vi "ziExample-Module-PIDAdvisor.vi"() -> ()   [LabVIEW 2009]
doc: "Control a Zurich instrument device via the LabOne Labview API. \nRequirements: Zurich Instruments HF2 +MF or UHFLI +MF \nPlease connect Signal input 1 and Signall Output 1.\nThis example shows how to configure a PID to regulate the output amplitude in order to achieve a constant input amplitude.\nThis example suggests a PID configuration via the PID advisor.\n\n© Zurich Instruments AG, www.zhinst.com"
uses:
  <instrlib>/Zurich Instruments LabOne/Public/ziTypeHandle.ctl
  <instrlib>/Zurich Instruments LabOne/Public/Modules/ziTypeModEnum.ctl
  <instrlib>/Zurich Instruments LabOne/Public/Modules/ziModSetValueBinary.vi
  <instrlib>/Zurich Instruments LabOne/Public/Configure/ziSetValueDouble.vi
  <instrlib>/Zurich Instruments LabOne/Public/Configure/ziSetValueDoubleArray.vi
  <instrlib>/Zurich Instruments LabOne/Public/Configure/ziGetValueString.vi
  <instrlib>/Zurich Instruments LabOne/Public/Modules/ziModSetValueDouble.vi
  <instrlib>/Zurich Instruments LabOne/Public/Modules/ziModSetValueDoubleArray.vi
  <instrlib>/Zurich Instruments LabOne/Public/Modules/ziModGetDoubleData.vi
  <instrlib>/Zurich Instruments LabOne/Public/Modules/ziModGetAdvisorData.vi
  <instrlib>/Zurich Instruments LabOne/Zurich Instruments LabOne.lvlib
panel:
  out "VALUE":dbl(graph)
  out "PID SHIFT":dbl(graph)
  out "demod/timeconstant":dbl
  out "Error Out":errorcluster
  out "Handle Out":T1 {"Handle" format="0x%08x"; "Conn" format="0x%08x"}
  in  "Calculate":bool
  in  "stop":bool
  out "PID ERROR":dbl(graph)
  in  "Address":string="DEV"
  in  "bw":dbl=100.0 caption="target BW (Hz)"
  in  "Mode":dbl(ring)=3.0 items=["P"=1.0, "I"=2.0, "PI"=3.0, "PID"=7.0, "PIDF"=15.0]
  out "i":dbl caption="I"
  out "p":dbl caption="P"
  out "dlimittimeconstant":dbl
  out "rate":dbl caption="Rate (Hz)"
  out "d":dbl caption="D"
  out "Step Response":cluster{"grid":dbl[], "r_avg":dbl[]}(graph)
  out "Bode Gain":cluster{"grid":dbl[], "r_avg":dbl[]}(graph)
  out "Bode Phase":cluster{"grid":dbl[], "r_avg":dbl[]}(graph)
  out "Selected Device":string
  # "ziExample-Module-PIDAdvisor.vi\nRequirements: UHFLI, HF2, MFLI +PID\nsee block diagram for VI description"
  # "Tested Devices:\n- UHFLI+PID \n- HF2+PID\n- MFLI+PID"
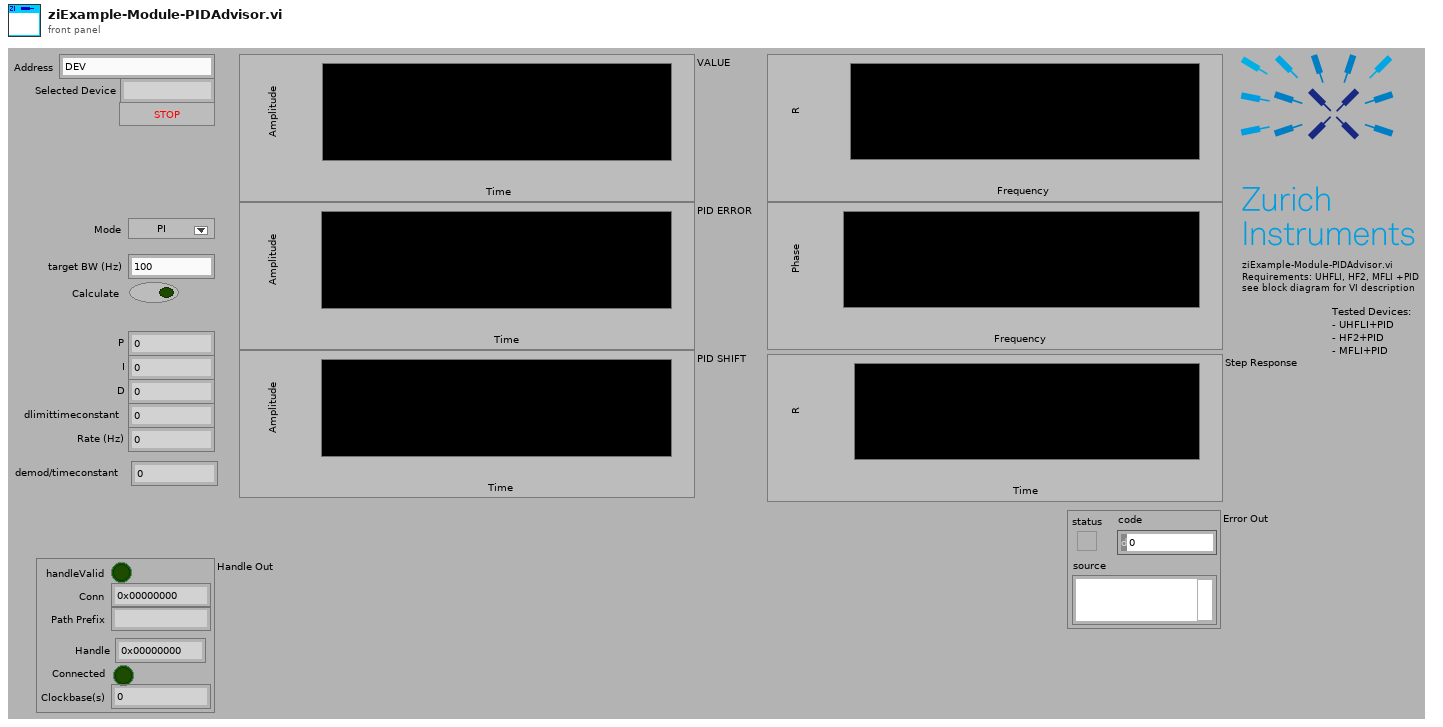
[diagram p1: front panel]
types:
  T1 = typedef "Zurich Instruments LabOne.lvlib/ziTypeHandle.ctl" = cluster{"handleValid":bool, "Conn":u64, "Path Prefix":string, "Handle":u64, "Connected":bool, "Clockbase(s)":dbl}
  T2 = typedef "Zurich Instruments LabOne.lvlib/ziTypeModEnum.ctl" = u16
  T3 = typedef "Zurich Instruments LabOne.lvlib/ziTypeModHandle.ctl" = cluster{"handleValid":bool, "Conn":u64, "ModHandle":u64, "moduleID":string, "Path Prefix":string}
  T4 = typedef "Zurich Instruments LabOne.lvlib/ziTypeModResults.ctl" = cluster{"PathArray":string[], "ValueType":T5, "NoOfResults":u64, "ziGenericHeader":T6[]}
  T5 = typedef "Zurich Instruments LabOne.lvlib/ziTypePollType.ctl" = enum16{"NONE", "DOUBLE_DATA", "INTEGER_DATA", "DEMOD_SAMPLE", "SCOPE_WAVE_HF2", "AUXIN_SAMPLE", "DIO_SAMPLE", "BYTE_ARRAY", "PWA_WAVE", "9", "10", "11", "12", "13", "14", "15", "TREE_CHANGE_DEPRI", "17", "ERROR", "19", "20", "21", "22", "23", "24", "25", "26", "27", "28", "29", "30", "31", "DOUBLE_DATA_TS", "INTEGER_DATA_TS", "34", "SCOPE_WAVE", "SCOPE_WAVE_EX", "37", "BYTE_ARRAY_TS", "39", "40", "41", "42", "43", "44", "45", "CNT_DATA", "47", "TREE_CHANGE", "49", "50", "51", "52", "53", "54", "55", "56", "57", "58", "59", "60", "61", "62", "63", "SWEEPER_DATA", "SPECTRUM_DATA", "ADVISOR_DATA", "VECTOR_DATA", "IMP_DATA"}
  T6 = typedef "Zurich Instruments LabOne.lvlib/ziTypeModGenericHeader.ctl" = cluster{"HeaderType":enum8{"HEADER_TYPE_NONE", "HEADER_TYPE_SWTRIGGER", "HEADER_TYPE_SWEEPER"}, "SampleFormat":u8, "SystemTime":timestamp, "CreatedTimeStamp":u64, "ChangedTimeStamp":u64, "Flags":u32, "ChunkSizeBytes":u64, "Name":string, "Status":u32, "GroupIndex":u32, "Color":u32, "ActiveRow":u32, "TriggerNumber":u64, "GridRows":u32, "GridCols":u32, "GridMode":u32, "GridOperation":u32, "GridDirection":u32, "GridRepetitions":u32, "GridColDelta":dbl, "GridColOffset":dbl, "GridRowDelta":dbl, "GridRowOffset":dbl, "Bandwidth":dbl, "Center":dbl, "Nenbw":dbl}
  T7 = typedef "Zurich Instruments LabOne.lvlib/ziTypeModAdvisorWave.ctl" = cluster{"timestamp":u64, "sampleCount":u64, "flags":u8, "sampleFormat":u8, "grid":dbl[], "x":dbl[], "y":dbl[]}
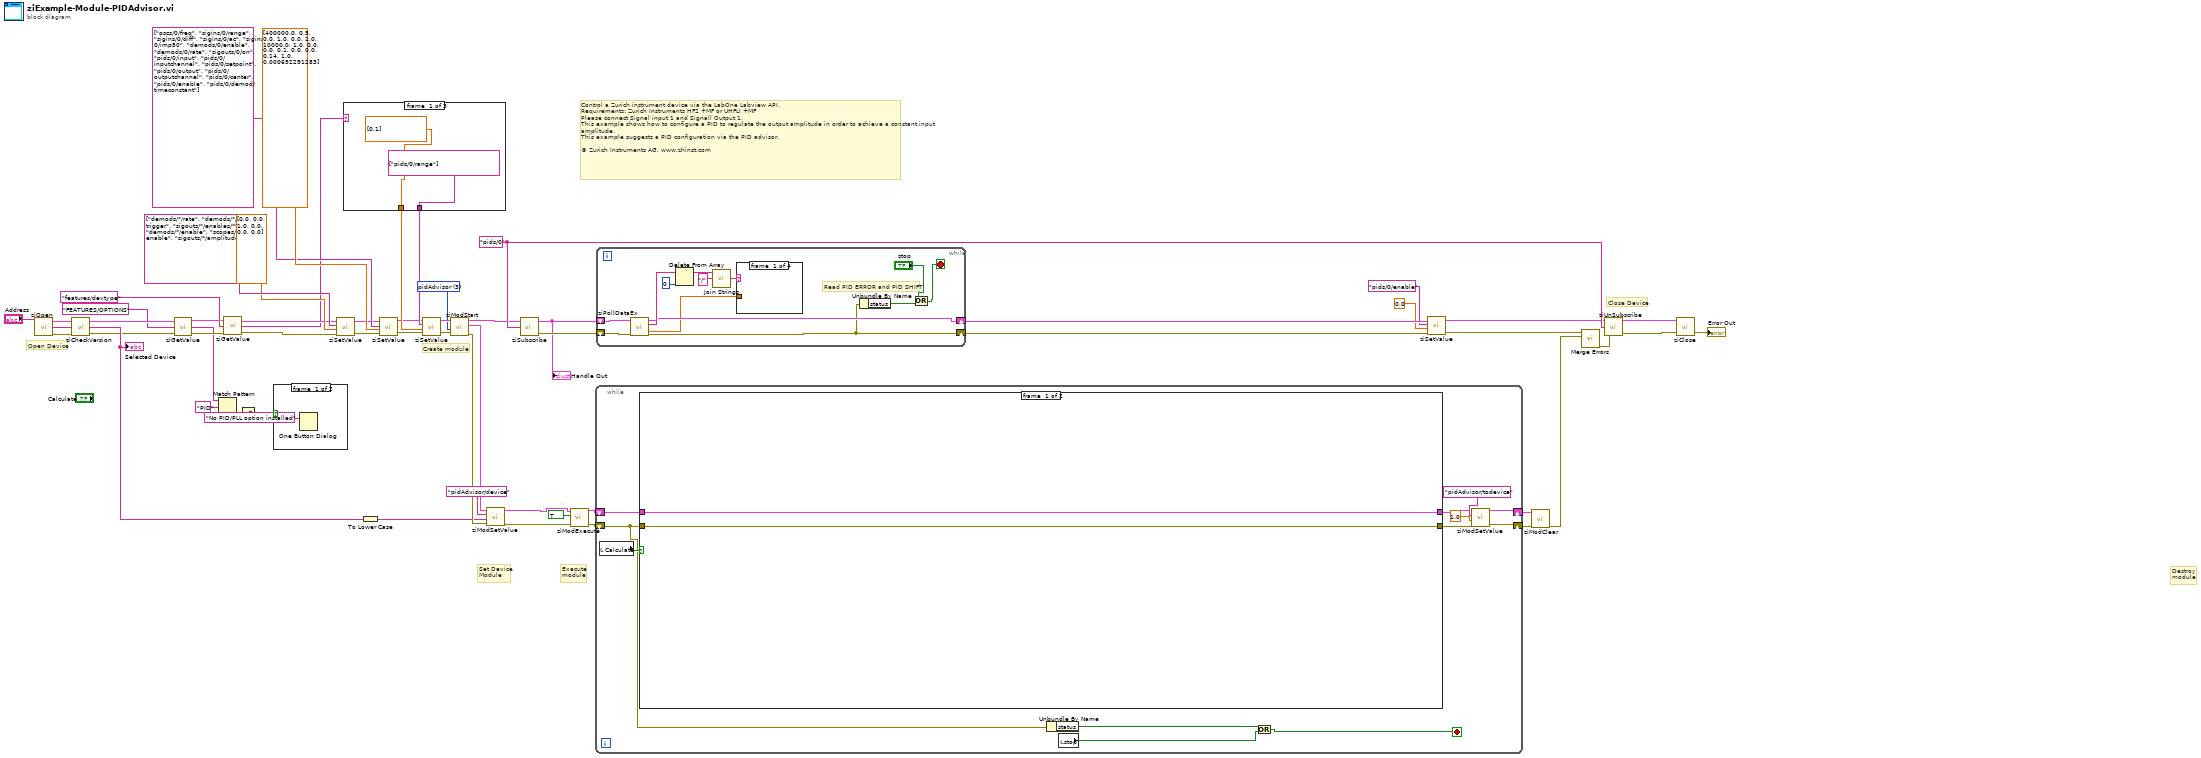
[diagram p0: block diagram]
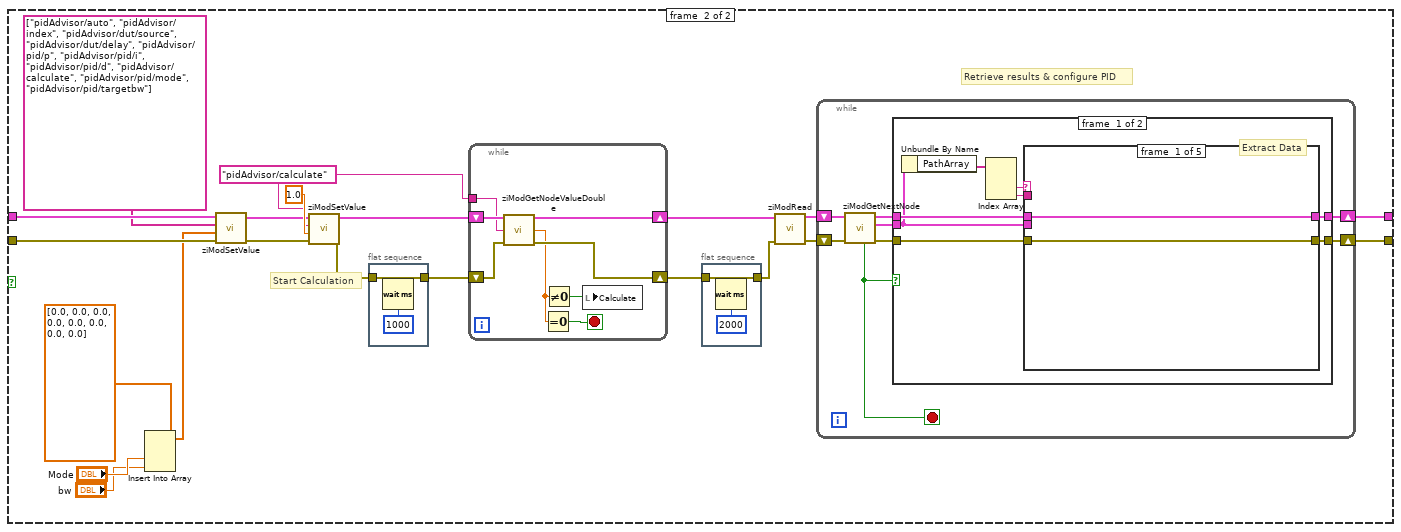
[diagram p3: hidden frame]
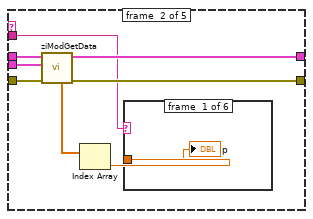
[diagram p4: hidden frame]
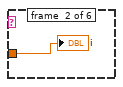
[diagram p5: hidden frame]
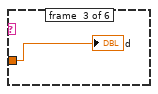
[diagram p6: hidden frame]
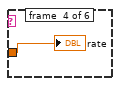
[diagram p7: hidden frame]
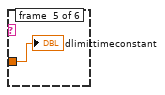
[diagram p8: hidden frame]
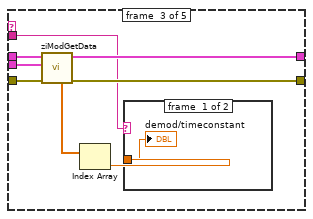
[diagram p10: hidden frame]
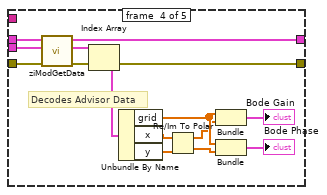
[diagram p12: hidden frame]
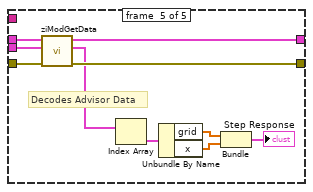
[diagram p13: hidden frame]
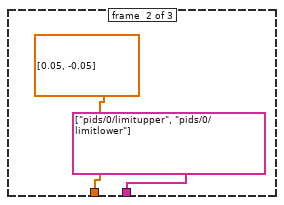
[diagram p15: hidden frame]
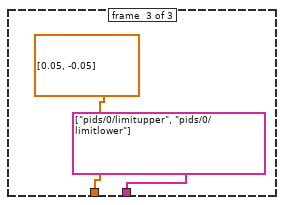
[diagram p16: hidden frame]
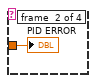
[diagram p17: hidden frame]
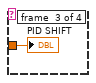
[diagram p18: hidden frame]
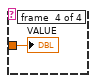
[diagram p19: hidden frame]
diagram:
  w15 = T2 3 items=["sweep", "scopeModule", "dataAcquisitionModule", "pidAdvisor", "awgModule", "impedanceModule", "multiDeviceSyncModule", "zoomFFT", "trigger", "deviceSettings", "record"] ("module Id")
  w38 = "pids/0" ("Path ()")
  # "Control a Zurich instrument device via the LabOne Labview API. \nRequirements: Zurich Instruments HF2 +MF or UHFLI +MF \nPlease connect Signal input 1 and Signall Output 1.\nThis example shows how to configure a PID to regulate the output amplitude in order to achieve a constant input amplitude.\nThis example suggests a PID configuration via the PID advisor.\n\n© Zurich Instruments AG, www.zhinst.com"
  # "Execute\nmodule"
  # "Set Device\nModule"
  # "Destroy\nmodule"
  # "Create module"
  # "Close Device"
  # "Open Device"
  n1 = call <instrlib>:"ziOpen.vi"("Address"="Address") -> ("Error Out"=w16:errorcluster, "Selected Device"=w36:string, "HandleOut"=w17:T1)  [unwired: 1 in, 2 out]
  "Selected Device" <- w36
  n2 = call <instrlib>:"ziCheckVersion.vi"("Handle In"=w17, "Error In"=w16) -> ("Handle Out"=w10:T1, "Error Out"=w9:errorcluster)  [unwired: 11 in, 1 out]
  n3 = call-poly <instrlib>:"ziGetValue.vi"("error in"=w9, "Path"="FEATURES/OPTIONS", "Handle In"=w10) -> ("error out"=w12:errorcluster, "Value"=w7:string, "Handle Out"=w11:T1)
  n4 = Match Pattern(string=w7, regular expression="PID") -> (offset past match=w13:i32)  [unwired: 1 in, 3 out]
  n5 = call-poly <instrlib>:"ziGetValue.vi"("error in"=w12, "Path"="features/devtype", "Handle In"=w11) -> ("error out"=w20:errorcluster, "Value"=w18:string, "Handle Out"=w21:T1)
  n6 = Greater Or Equal To 0?(x=w13) -> (x >= 0?=w1:bool)
  n7 = case shown="True" w1 {
    frame #0 {
      n8 = One Button Dialog(message="No PID/PLL option installed") -> ()  [unwired: 1 in, 1 out]
    }
    frame #1 {
    }
  }
  n9 = call-poly <instrlib>:"ziSetValue.vi"("Error In"=w20, "Values"=dbl[] [0.0, 0.0, 1.0, 0.0, 0.0, 0.0], "Paths"=string[] ["demods/*/rate", "demods/*/trigger", "sigouts/*/enables/*", "demods/*/enable", "scopes/*/enable", "sigouts/*/amplitudes/*"], "Handle In"=w21) -> ("Error Out"=w22:errorcluster, "Handle Out"=w23:T1)  [unwired: 1 in]
  n10 = case shown="\"MFIA\", \"MFLI\"" w18 {
    tunnel: [dbl[] [0.1] dbl[] [0.05, -0.05] dbl[] [0.05, -0.05]] -> w43
    tunnel: [string[] ["pids/0/range"] string[] ["pids/0/limitupper", "pids/0/limitlower"] string[] ["pids/0/limitupper", "pids/0/limitlower"]] -> w42
    frame #0 {
    }
    frame #1 {
    }
    frame #2 {
    }
  }
  n11 = To Lower Case(string=w36) -> (all lower case string=w35:string)
  n12 = call-poly <instrlib>:"ziSetValue.vi"("Error In"=w22, "Values"=dbl[] [400000.0, 0.5, 0.0, 1.0, 0.0, 1.0, 10000.0, 1.0, 0.0, 0.0, 0.1, 0.0, 0.0, 0.14, 1.0, 0.000692291283], "Paths"=string[] ["oscs/0/freq", "sigins/0/range", "sigins/0/diff", "sigins/0/ac", "sigins/0/imp50", "demods/0/enable", "demods/0/rate", "sigouts/0/on", "pids/0/input", "pids/0/inputchannel", "pids/0/setpoint", "pids/0/output", "pids/0/outputchannel", "pids/0/center", "pids/0/enable", "pids/0/demod/timeconstant"], "Handle In"=w23) -> ("Error Out"=w27:errorcluster, "Handle Out"=w28:T1)  [unwired: 1 in]
  n13 = call-poly <instrlib>:"ziSetValue.vi"("Error In"=w27, "Values"=w43, "Paths"=w42, "Handle In"=w28) -> ("Error Out"=w55:errorcluster, "Handle Out"=w56:T1)  [unwired: 1 in]
  n14 = call <instrlib>:"ziModStart.vi"("Error In"=w55, "module Id"=w15, "Handle In"=w56) -> ("Error Out"=w46:errorcluster, "ModHandle Out"=w52:T3, "Handle Out"=w19:T1)  [unwired: 6 in]
  n15 = call-poly <instrlib>:"ziModSetValue.vi"("Error In"=w46, "Data"=w35, "Path"="pidAdvisor/device", "ModHandle In"=w52) -> ("Error Out"=w5:errorcluster, "ModHandle Out"=w6:T3)  [unwired: 6 in]
  n16 = call <instrlib>:"ziSubscribe.vi"("Path ()"=w38, "Handle In"=w19) -> ("error out"=w53:errorcluster, "Handle Out"=w47:T1)  [unwired: 2 in]
  "Handle Out" <- w47
  n17 = call <instrlib>:"ziModExecute.vi"("Error In"=w5, "Modal (F)"=TRUE ("Modal"), "ziModHandle In"=w6) -> ("Error Out"=w51:errorcluster, "ziModHandle Out"=w48:T3)  [unwired: 5 in, 1 out]
  n18 = while {
    shift-right: [w70] -> w3
    shift-left: w48 -> [w75]
    shift-right: [w69] -> w4
    shift-left: w51 -> [w67]
    stop <- w64 stop-if-true
    n19 = local read "Calculate"() -> (w74:bool)
    n20 = case shown="True" w74 {
      tunnel: w75 -> [w76 w92]
      tunnel: w67 -> [w77 w93]
      tunnel: [w77 w85] -> w68
      tunnel: [w76 w86] -> w71
      frame #0 {
      }
      frame #1 {
        w79 = "pidAdvisor/calculate" ("Path")
        # "Extract Data"
        # "Retrieve results & configure PID"
        # "Start Calculation"
        n21 = Insert Into Array(array=dbl[] [0.0, 0.0, 0.0, 0.0, 0.0, 0.0, 0.0, 0.0], new element #1="Mode", new element #2="bw") -> (w80:dbl[])  [unwired: 1 in]
        n22 = call-poly <instrlib>:"ziModSetValue.vi"("Error In"=w93, "Values"=w80, "Paths"=string[] ["pidAdvisor/auto", "pidAdvisor/index", "pidAdvisor/dut/source", "pidAdvisor/dut/delay", "pidAdvisor/pid/p", "pidAdvisor/pid/i", "pidAdvisor/pid/d", "pidAdvisor/calculate", "pidAdvisor/pid/mode", "pidAdvisor/pid/targetbw"], "ModHandle In"=w92) -> ("Error Out"=w78:errorcluster, "ModHandle Out"=w81:T3)  [unwired: 6 in]
        n23 = call-poly <instrlib>:"ziModSetValue.vi"("Error In"=w78, "Value"=1.0, "Path"=w79, "ModHandle In"=w81) -> ("Error Out"=w91:errorcluster, "ModHandle Out"=w96:T3)  [unwired: 6 in]
        n24 = flat-sequence {
          tunnel: [w102] -> w90
          tunnel: w91 -> [w102]
          frame #0 {
            n25 = Wait (ms)(milliseconds to wait=u32 1000) -> ()  [unwired: 1 out]
          }
        }
        n26 = while {
          shift-right: [w172] -> w97
          shift-left: w96 -> [w175]
          shift-right: [w173] -> w88
          shift-left: w90 -> [w176]
          tunnel: w79 -> [w174]
          stop <- w171 stop-if-true
          n27 = call <instrlib>:"ziModGetNodeValueDouble.vi"("ModHandle In"=w175, "Path"=w174, "error in"=w176) -> ("ModHandle Out"=w172:T3, "Value"=w169:dbl, "error out"=w173:errorcluster)  [unwired: 10 in]
          n28 = Equal To 0?(x=w169) -> (x = 0?=w171:bool)
          n29 = Not Equal To 0?(x=w169) -> (x != 0?=w170:bool)
          n30 = local write "Calculate"(w170) -> ()
        }
        n31 = flat-sequence {
          tunnel: w88 -> [w99]
          tunnel: [w99] -> w87
          frame #0 {
            n32 = Wait (ms)(milliseconds to wait=u32 2000) -> ()  [unwired: 1 out]
          }
        }
        n33 = call <instrlib>:"ziModRead.vi"("error in"=w87, "ziModHandle In"=w97) -> ("error out"=w94:errorcluster, "ziModHandle Out"=w95:T3)  [unwired: 8 in]
        n34 = while {
          shift-right: [w104] -> w86
          shift-left: w95 -> [w109]
          shift-right: [w103] -> w85
          shift-left: w94 -> [w110]
          stop <- w105 stop-if-true
          n35 = call <instrlib>:"ziModGetNextNode.vi"("Error In"=w110, "ModHandle In"=w109) -> ("Error Out"=w107:errorcluster, "ModResults"=w106:T4, "ModHandle Out"=w108:T3, "NoData"=w105:bool)  [unwired: 6 in]
          n36 = case shown="False" w105 {
            tunnel: w108 -> [w118 w168]
            tunnel: w107 -> [w117 w167]
            tunnel: w106 -> [w114 _]
            tunnel: [w116 w168] -> w104
            tunnel: [w115 w167] -> w103
            frame #0 {
              n37 = Unbundle By Name(w114) -> ("PathArray"=w113:string[])
              n38 = Index Array(array=w113) -> (element #2=w111:string, element #3=w112:string)  [unwired: 3 in, 1 out]
              n39 = case shown="Default" w111 {
                tunnel: w118 -> [w120 w128 w141 w155 w165]
                tunnel: w114 -> [_ w127 w140 w156 w166]
                tunnel: w117 -> [w119 w126 w139 w154 w164]
                tunnel: [w119 w123 w136 w153 w163] -> w115
                tunnel: [w120 w125 w138 w152 w162] -> w116
                tunnel: w112 -> [_ w122 w135 _ _]
                frame #0 {
                }
                frame #1 {
                  n40 = call-poly <instrlib>:"ziModGetData.vi"("Error In"=w126, "ModResults"=w127, "ModHandle In"=w128) -> ("Error Out"=w123:errorcluster, "ModHandle Out"=w125:T3, "Value"=w121:dbl[])  [unwired: 4 in, 2 out]
                  n41 = Index Array(array=w121) -> (element=w124:dbl)  [unwired: 1 in]
                  n42 = case shown="\"d\"" w122 {
                    tunnel: w124 -> [w129 w130 w131 w132 w133 _]
                    frame #0 {
                      "p" <- w129
                    }
                    frame #1 {
                      "i" <- w130
                    }
                    frame #2 {
                      "d" <- w131
                    }
                    frame #3 {
                      "rate" <- w132
                    }
                    frame #4 {
                      "dlimittimeconstant" <- w133
                    }
                    frame #5 {
                    }
                  }
                }
                frame #2 {
                  n43 = call-poly <instrlib>:"ziModGetData.vi"("Error In"=w139, "ModResults"=w140, "ModHandle In"=w141) -> ("Error Out"=w136:errorcluster, "ModHandle Out"=w138:T3, "Value"=w134:dbl[])  [unwired: 4 in, 2 out]
                  n44 = Index Array(array=w134) -> (element=w137:dbl)  [unwired: 1 in]
                  n45 = case shown="\"timeconstant\"" w135 {
                    tunnel: w137 -> [w142 _]
                    frame #0 {
                      "demod/timeconstant" <- w142
                    }
                    frame #1 {
                    }
                  }
                }
                frame #3 {
                  # "Decodes Advisor Data"
                  n46 = call-poly <instrlib>:"ziModGetData.vi"("Error In"=w154, "ModResults"=w156, "ModHandle In"=w155) -> ("Error Out"=w153:errorcluster, "AdvisorData Out"=w150:T7[], "ModHandle Out"=w152:T3)  [unwired: 6 in]
                  n47 = Index Array(array=w150) -> (element=w151:T7)  [unwired: 1 in]
                  n48 = Unbundle By Name(w151) -> ("grid"=w147:dbl[], "x"=w143:dbl[], "y"=w144:dbl[])
                  n49 = Re/Im To Polar(2:w144, 3:w143) -> (0:w145:dbl[], 1:w146:dbl[])
                  n50 = Bundle("grid"=w147, w146) -> (→"Bode Gain":cluster{"grid":dbl[], dbl[]})  [unwired: 1 in]
                  n51 = Bundle("grid"=w147, w145) -> (→"Bode Phase":cluster{"grid":dbl[], dbl[]})  [unwired: 1 in]
                }
                frame #4 {
                  # "Decodes Advisor Data"
                  n52 = call-poly <instrlib>:"ziModGetData.vi"("Error In"=w164, "ModResults"=w166, "ModHandle In"=w165) -> ("Error Out"=w163:errorcluster, "AdvisorData Out"=w160:T7[], "ModHandle Out"=w162:T3)  [unwired: 6 in]
                  n53 = Index Array(array=w160) -> (element=w161:T7)  [unwired: 1 in]
                  n54 = Unbundle By Name(w161) -> ("grid"=w159:dbl[], "x"=w158:dbl[])
                  n55 = Bundle("grid"=w159, "x"=w158) -> (→"Step Response":cluster{"grid":dbl[], "x":dbl[]})  [unwired: 1 in]
                }
              }
            }
            frame #1 {
              (unwired) FALSE
            }
          }
        }
      }
    }
    n56 = Unbundle By Name(w67) -> ("status"=w66:bool)
    n57 = local read "stop"() -> (w65:bool)
    n58 = Or(x=w66, y=w65) -> (x .or. y?=w64:bool)
    n59 = call-poly <instrlib>:"ziModSetValue.vi"("Error In"=w68, "Value"=1.0, "Path"="pidAdvisor/todevice", "ModHandle In"=w71) -> ("Error Out"=w69:errorcluster, "ModHandle Out"=w70:T3)  [unwired: 6 in]
  }
  n60 = while {
    shift-right: [w182] -> w33
    shift-left: w47 -> [w189]
    shift-right: [w180] -> w34
    shift-left: w53 -> [w188]
    stop <- w177 stop-if-true
    # "Read PID ERROR and PID SHIFT"
    n61 = call <instrlib>:"ziPollDataEx.vi"("error in"=w188, "Handle In"=w189) -> ("error out"=w180:errorcluster, "PathArray"=w186:string[], "Handle Out"=w182:T1, "Value Double"=w181:dbl)  [unwired: 2 in, 4 out]
    n62 = Delete From Array(array=w186, index=0) -> (array with subset deleted=w185:string[])  [unwired: 1 in, 1 out]
    n63 = call <vilib>:"Join Strings.vi"("Separator (,)"="/" ("delimiter (Tab)"), "Strings In"=w185) -> ("String"=w183:string)  [unwired: 1 in]
    n64 = case shown="\"PIDS/0/STREAM/VALUE\", \"PIDS/0/VALUE\"" w183 {
      tunnel: w181 -> [_ w190 w191 w192]
      frame #0 {
      }
      frame #1 {
        "PID ERROR" <- w190
      }
      frame #2 {
        "PID SHIFT" <- w191
      }
      frame #3 {
        "VALUE" <- w192
      }
    }
    n65 = Unbundle By Name(w180) -> ("status"=w179:bool)
    n66 = Or(x="stop", y=w179) -> (x .or. y?=w177:bool)
  }
  n67 = call-poly <instrlib>:"ziSetValue.vi"("Error In"=w34, "Value"=0.0, "Path"="pids/0/enable", "Handle In"=w33) -> ("Error Out"=w26:errorcluster, "Handle Out"=w32:T1)  [unwired: 1 in]
  n68 = call <instrlib>:"ziModClear.vi"("Error In"=w4, "ziModHandle In"=w3) -> ("Error Out"=w2:errorcluster)  [unwired: 7 in, 1 out]
  n69 = call <vilib>:"Merge Errors.vi"("error in 2 (no error)"=w2, "error in 1 (no error)"=w26) -> ("error out"=w24:errorcluster)  [unwired: 5 in]
  n70 = call <instrlib>:"ziUnSubscribe.vi"("error in"=w24, "Path (\"/\")"=w38, "Handle in"=w32) -> ("error out"=w25:errorcluster, "Handle out"=w37:T1)  [unwired: 1 in]
  n71 = call <instrlib>:"ziClose.vi"("Error In"=w25, "Handle In"=w37) -> ("Error Out"=→"Error Out":errorcluster)  [unwired: 2 in, 1 out]
